vi "Open Hardware.vi"(8 "error in (no error)":errorcluster, 11 "Instrument.Template in":refnum<class "Instrument.LN2.lvclass">) -> (0 "error out":errorcluster, 3 "Instrument.Template out":refnum<class "Instrument.LN2.lvclass">)   [LabVIEW 2019, in "Instrument.LN2.lvclass"]
uses:
  Instrument.LN2.lvclass
  C:/Program Files (x86)/National Instruments/LabVIEW 2019/user.lib/LevyLab/Instrument Framework/SMOs/Instrument/Instrument.lvclass
  <userlib>/LevyLab/Instrument Framework/SMOs/Instrument/Instrument.lvclass/Instrument.ctl
  Instrument.LN2.lvclass/Instrument.LN2.ctl
  <userlib>/LevyLab/Instrument Framework/Instrument Types/VSource/Instrument.VSource.lvclass
  <userlib>/LevyLab/Instrument Framework/SMOs/Instrument/Instrument.lvclass
  <vilib>/Instr/_visa.llb/VISA Configure Serial Port (Instr).vi
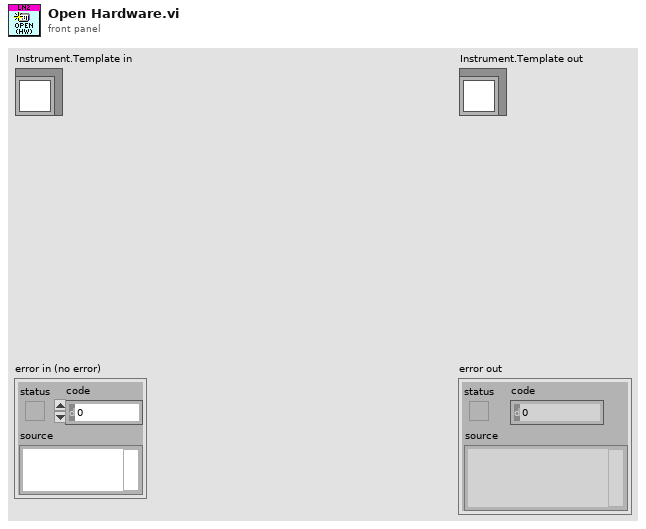
[diagram p1: front panel]
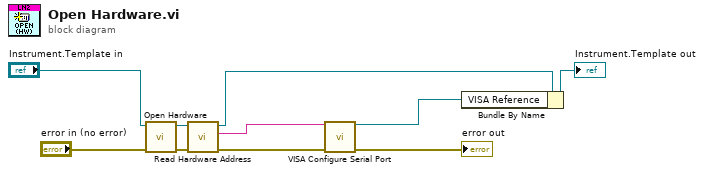
[diagram p0: block diagram]
diagram:
  n1 = call-parent "Open Hardware.vi"("error in (no error)"="error in (no error)", "Instrument in"="Instrument.Template in") -> ("error out"=w7:errorcluster, "Instrument out"=w8:refnum<class "Instrument.LN2.lvclass">)  [unwired: 8 in]
  n2 = call <userlib>:"Read Hardware Address.vi"("error in (no error)"=w7, "Instrument in"=w8) -> ("error out"=w3:errorcluster, "Address"=w1:string, "Instrument out"=w6:refnum<class "Instrument.LN2.lvclass">)  [unwired: 7 in]
  n3 = call-poly "VISA Configure Serial Port"("VISA resource name"=w1, "error in (no error)"=w3) -> ("VISA resource name out"=w2:refnum<visa-resource-name>, "error out"=→"error out":errorcluster)  [unwired: 12 in]
  n4 = Bundle By Name(cluster=w6, "VISA Reference"=w2) -> (→"Instrument.Template out":refnum<class "Instrument.LN2.lvclass">)
